vi "Generate VC Sine Wave.vi"(6 "Counter":i32, 7 "Period (us)":i64, 9 "offset (V)":dbl, 10 "amplitude (V)":dbl, 11 "frequency (kHz)":dbl) -> (3 "V":dbl)   [LabVIEW 2018]
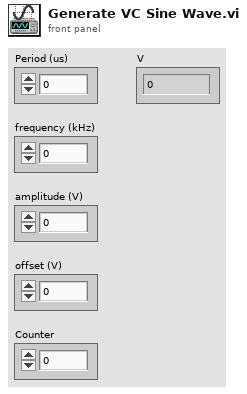
[diagram p1: front panel]
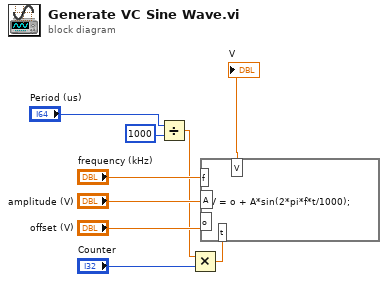
[diagram p0: block diagram]
diagram:
  n1 = Divide(x="Period (us)", y=1000) -> (x/y=w3:dbl)
  n2 = Multiply(x=w3, y="Counter") -> (x*y=w7:dbl)
  n3 = formula code="V = o + A*sin(2*pi*f*t/1000);"("f"="frequency (kHz)", "A"="amplitude (V)", "t"=w7, "o"="offset (V)") -> ("V"=→"V":dbl)
